vi "Get AdsSymbolInfoCollection DVR.vi"(8 "error in (no error)":errorcluster, 11 "TwinCAT ADS in":refnum<class "TwinCAT ADS.lvclass">) -> (0 "error out":errorcluster, 2 "AdsSymbolInfoCollection DVR":refnum<data-value>, 3 "TwinCAT ADS out":refnum<class "TwinCAT ADS.lvclass">)   [LabVIEW 2018, in "TwinCAT ADS.lvclass"]
uses:
  TwinCAT ADS.lvclass
  TwinCAT.Ads
  TwinCAT ADS.lvclass/TwinCAT ADS.ctl
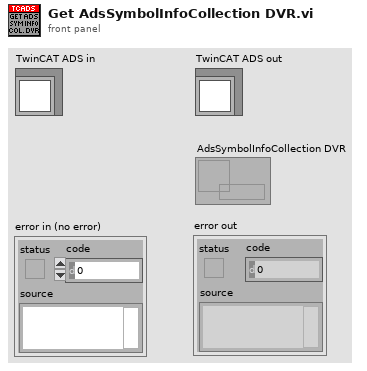
[diagram p1: front panel]
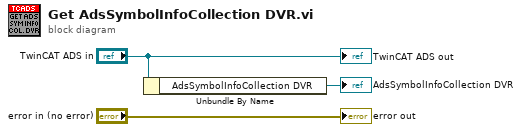
[diagram p0: block diagram]
diagram:
  n1 = Unbundle By Name("TwinCAT ADS in") -> ("AdsSymbolInfoCollection DVR"=→"AdsSymbolInfoCollection DVR":refnum<data-value>)
  "error out" <- "error in (no error)"
  "TwinCAT ADS out" <- "TwinCAT ADS in"
